vi "Do.vi"(8 "error in (no error)":errorcluster, 10 "Actor in":refnum<class "Actor.lvclass">, 11 "Udpate Task Display Name Msg in":refnum<class "Udpate Task Display Name Msg.lvclass">) -> (0 "error out":errorcluster, 2 "Actor out":refnum<class "Actor.lvclass">)   [LabVIEW 2017, in "Task Setting Editor.lvlib" / "Udpate Task Display Name Msg.lvclass"]
doc: "This VI delivers the message to the actor by calling the appropriate method(s) on the actor."
uses:
  Udpate Task Display Name Msg.lvclass
  <vilib>/ActorFramework/Actor/Actor.lvclass
  Udpate Task Display Name Msg.lvclass/Udpate Task Display Name Msg.ctl
  Task Setting Editor/Task Setting Editor.lvclass
  C:/Program Files (x86)/National Instruments/LabVIEW 2017/vi.lib/ActorFramework/Actor/Actor.lvclass
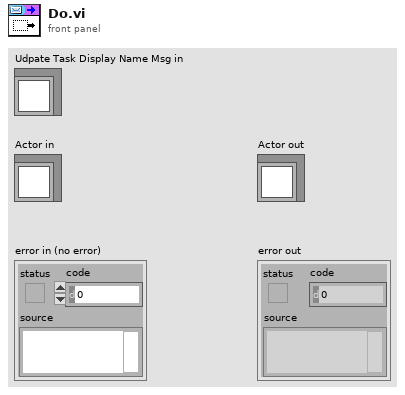
[diagram p1: front panel]
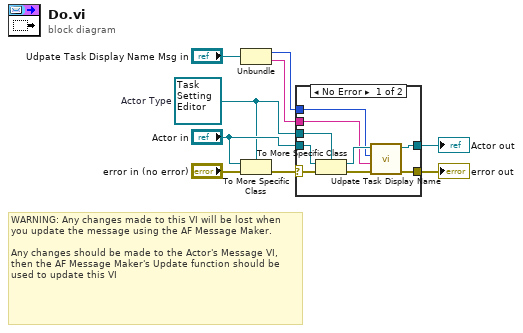
[diagram p0: block diagram]
diagram:
  w4 = refnum<class "Task Setting Editor.lvclass"> refnum  # Actor Type
  # "WARNING: Any changes made to this VI will be lost when you update the message using the AF Message Maker.\n\nAny changes should be made to the Actor's Message VI, then the AF Message Maker's Update function should be used to update this VI"
  n1 = Unbundle("Udpate Task Display Name Msg in") -> (w3:i32, w2:string)
  n2 = To More Specific Class(target class=w4, reference="Actor in", error in="error in (no error)") -> (error out=w8:errorcluster)  [unwired: 1 out]
  n3 = case shown="No Error" w8 {
    selector: w8 -> [w18 w20]
    tunnel: [w13 w20] -> w7
    tunnel: [w12 w19] -> w6
    tunnel: "Actor in" -> [w17 w19]
    tunnel: w4 -> [w16 _]
    tunnel: w3 -> [w11 _]
    tunnel: w2 -> [w10 _]
    frame No Error {
      n4 = To More Specific Class ("Actor Cast")(target class=w16, reference=w17, error in=w18) -> (specific class reference=w15:refnum<class "Task Setting Editor.lvclass">, error out=w14:errorcluster)
      n5 = call "Udpate Task Display Name.vi"("error in (no error)"=w14, "Display Name"=w10, "Task"=w11, "Task Setting Editor in"=w15) -> ("error out"=w13:errorcluster, "Task Setting Editor out"=w12:refnum<class "Task Setting Editor.lvclass">)  [unwired: 6 in]
    }
    frame Error {
    }
  }
  "error out" <- w7
  "Actor out" <- w6
